vi "Main.vi"(11 "Error in":errorcluster) -> (15 "Error out":errorcluster)   [LabVIEW 2020, in "File explorer 2.0.lvlib"]
doc: "This VI is the expanded implementation of file explorer here this has additional features of adding and getting folder data and copying the selected files form one location to another location"
uses:
  File explorer 2.0.lvlib
  Typedefs/Data Cluster.ctl
  <vilib>/Utility/miscctls.llb/LVPositionTypeDef.ctl
  Typedefs/Queue operations.ctl
panel:
  in  "Stop":bool
  in  "Search":string
  in  "Copy":bool
  in  "Operation":bool
  in  "File input":path
  in  "File system":string(tree)
  out "File details":string
  # "FILE EXPLORER 2.0"
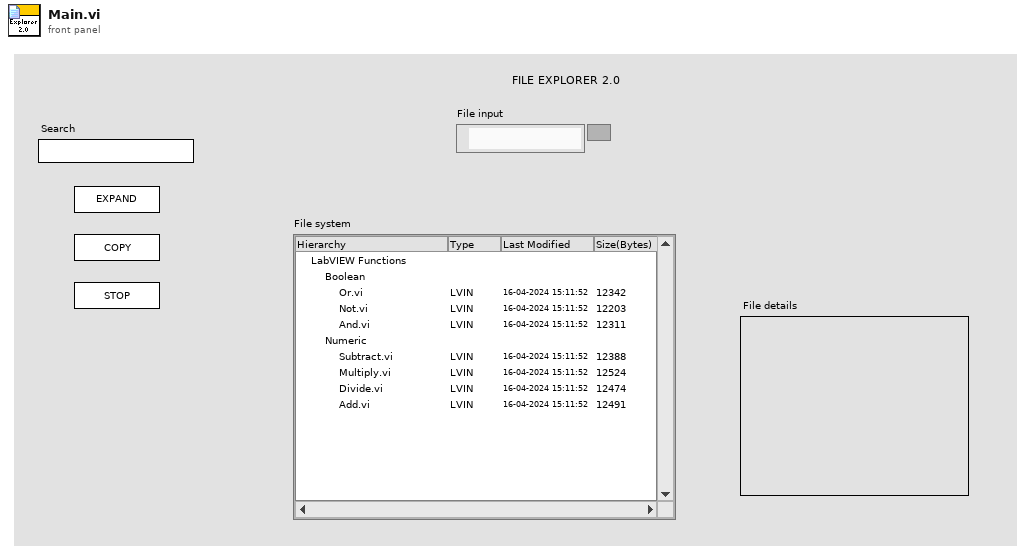
[diagram p1: front panel]
types:
  T1 = typedef "File explorer 2.0.lvlib/Queue operations.ctl" = enum16{"Create", "Enqueue", "Enstack", "Dequeue", "Flush", "Release"}
  T2 = typedef "File explorer 2.0.lvlib/Data Cluster.ctl" = cluster{"Copy":bool, "Operation":bool, "File input":path, "Search":string, "File details":string, "Folder":string[], "Position":T3, "Selected Files":string[], "Reverse":bool}
  T3 = typedef "LVPositionTypeDef.ctl" = cluster{"Left":i32, "Top":i32}
  T4 = typedef "LVPoint32TypeDef.ctl" = cluster{"Horizontal":i32, "Vertical":i32}
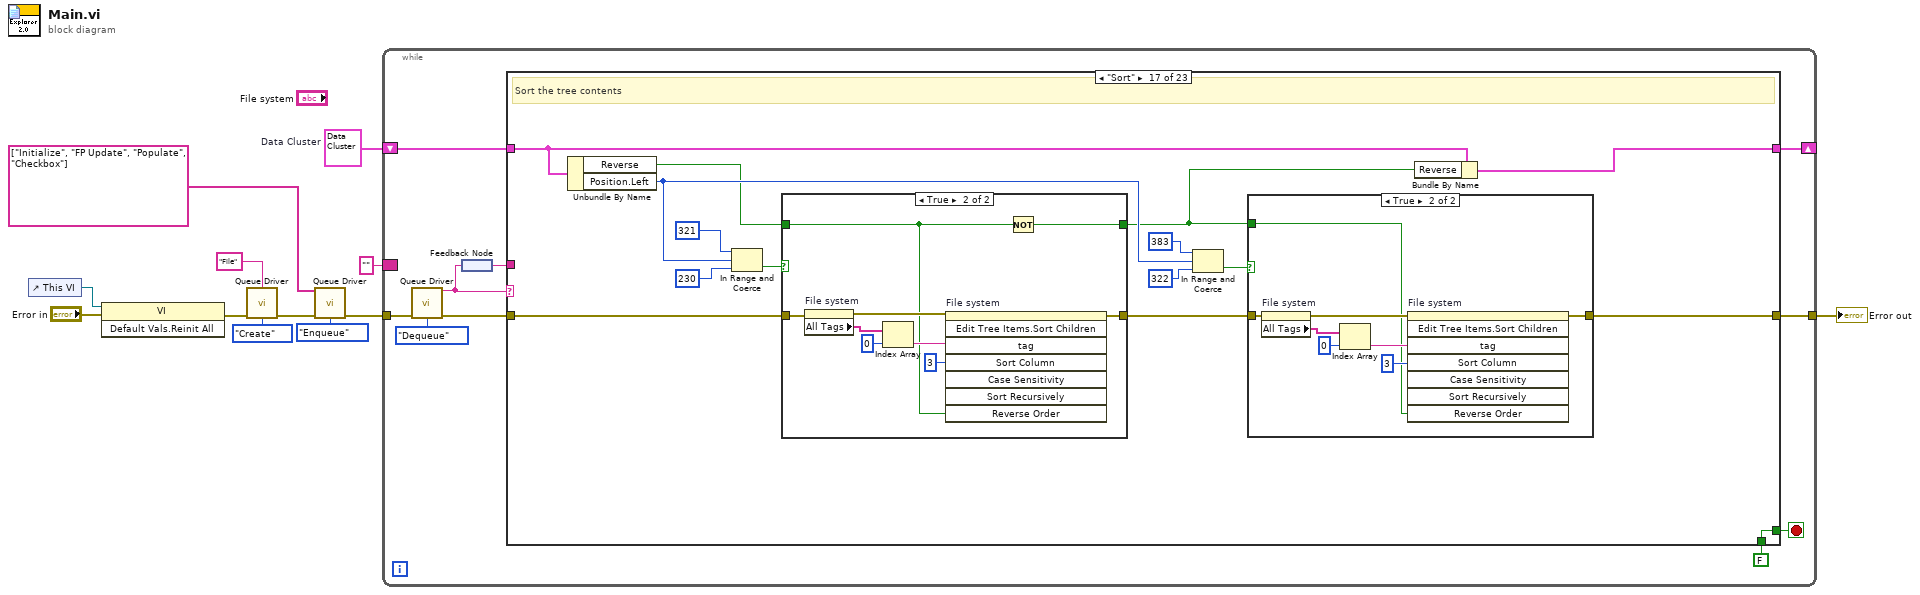
[diagram p0: block diagram]
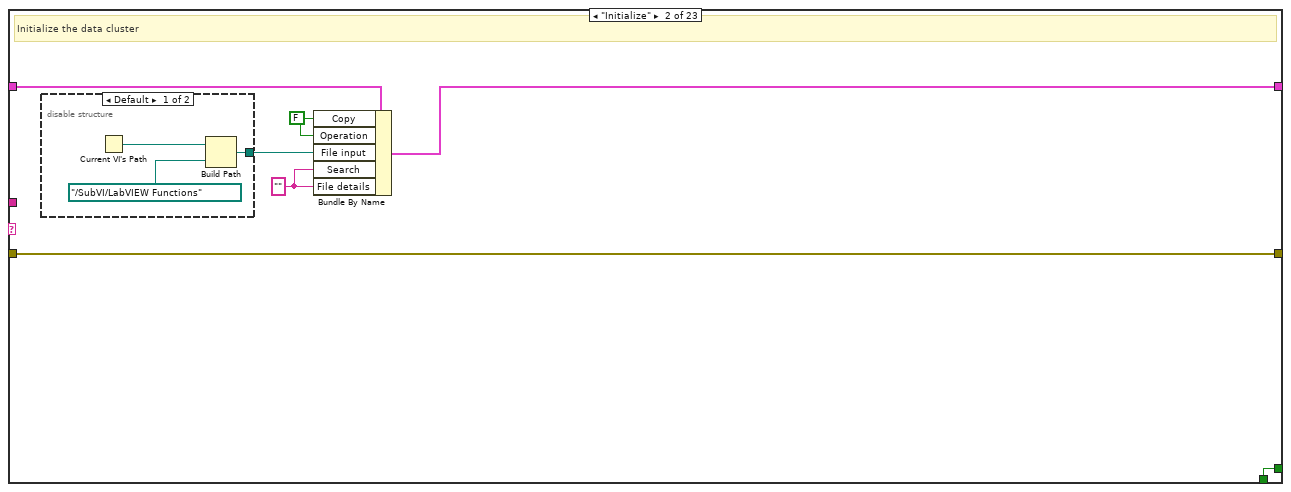
[diagram p3: hidden frame]
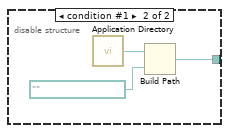
[diagram p4: hidden frame]
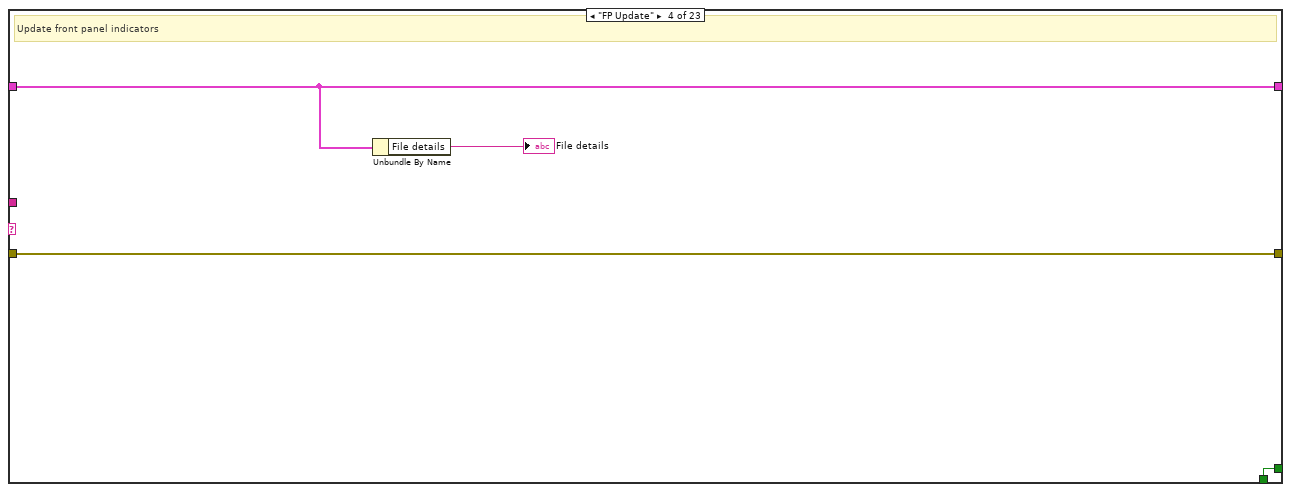
[diagram p6: hidden frame]
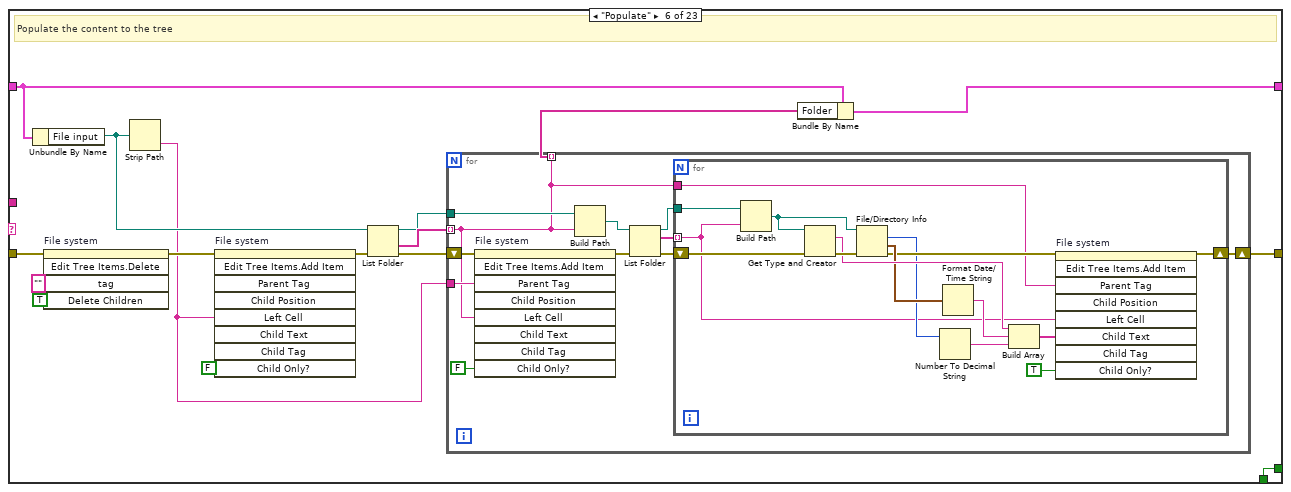
[diagram p8: hidden frame]
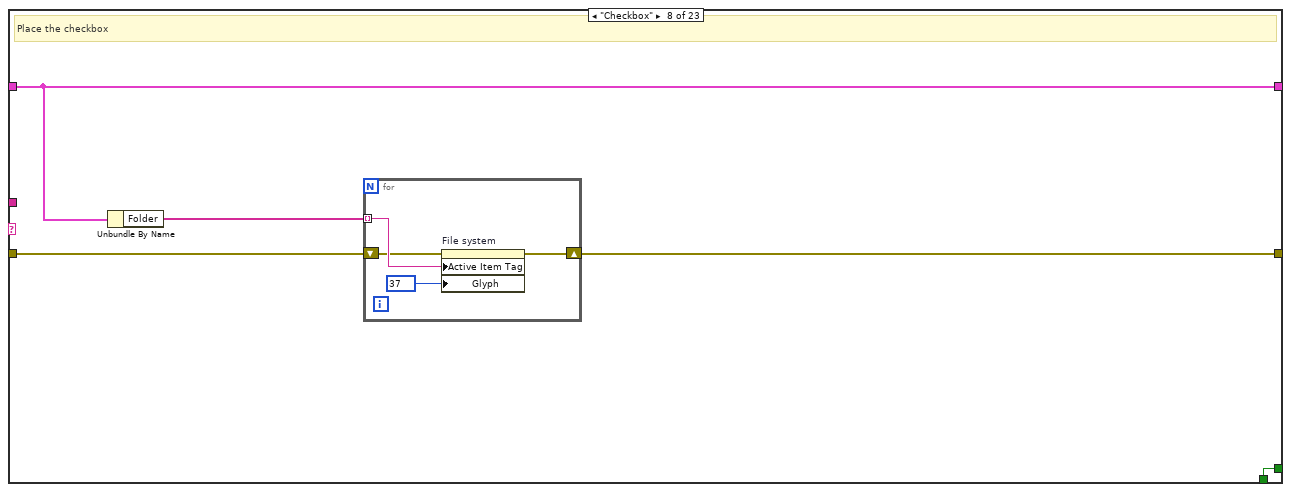
[diagram p10: hidden frame]
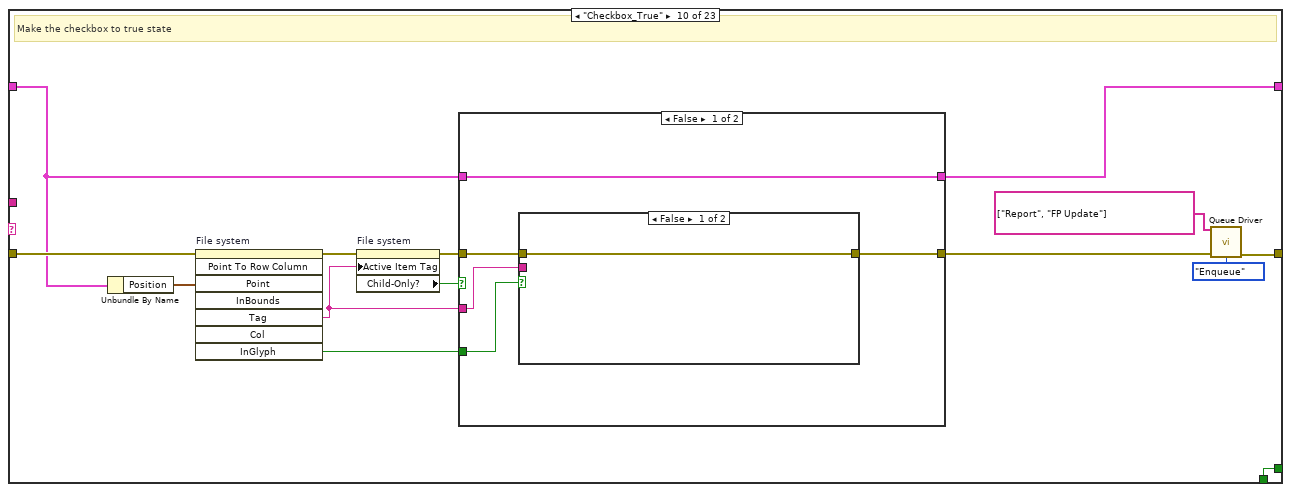
[diagram p12: hidden frame]
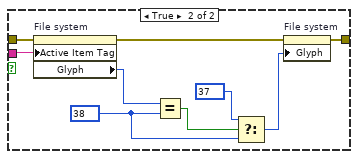
[diagram p13: hidden frame]
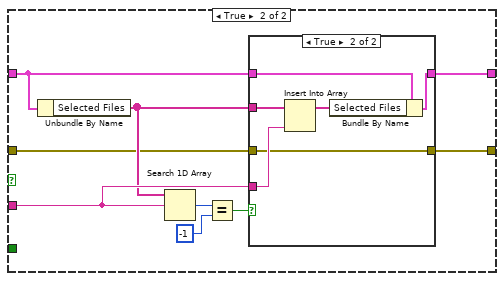
[diagram p14: hidden frame]
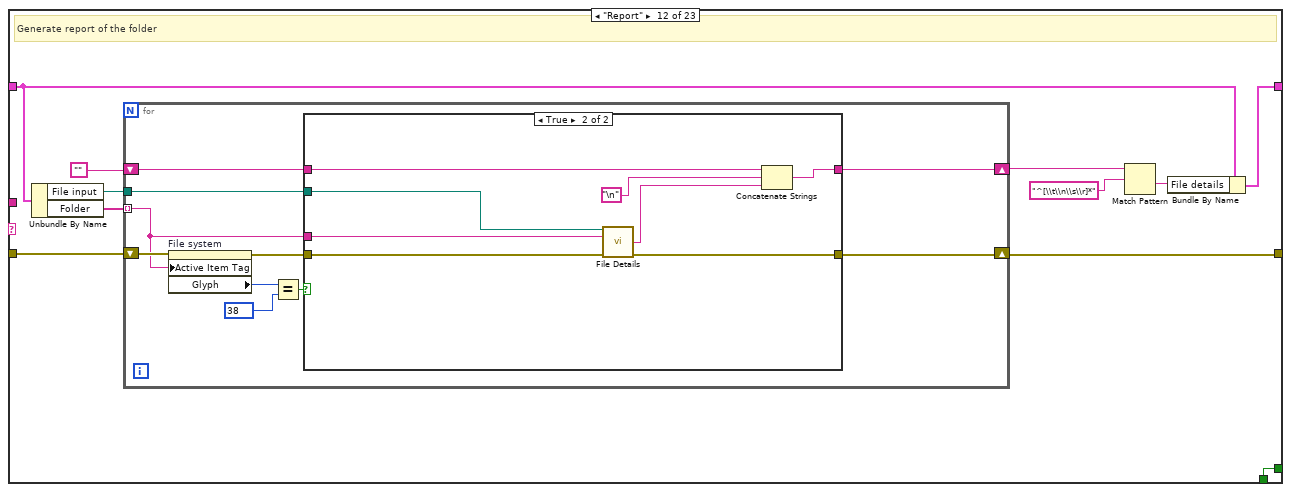
[diagram p17: hidden frame]
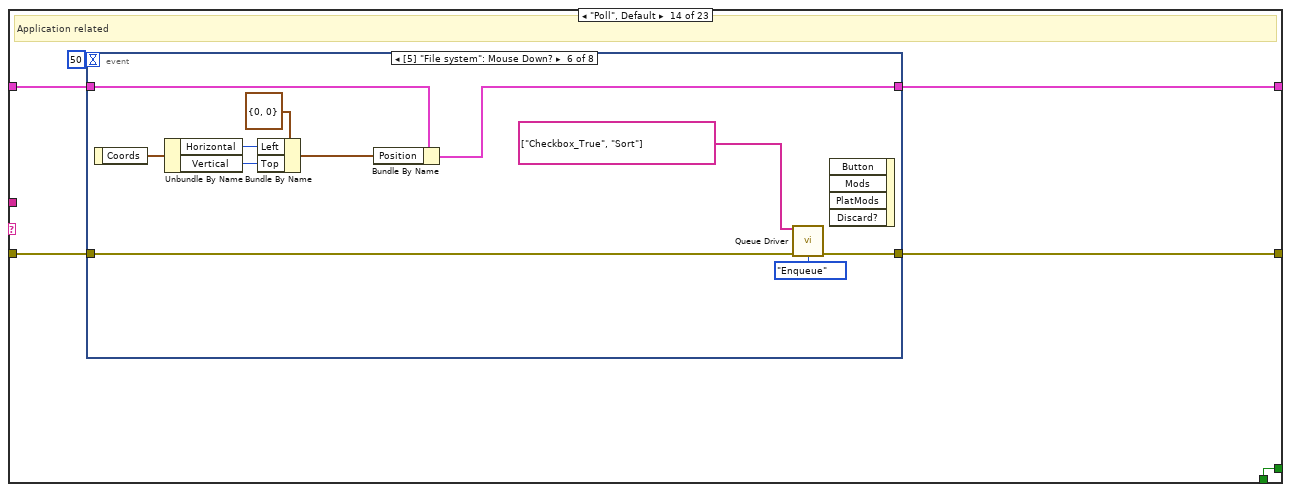
[diagram p20: hidden frame]
diagram:
  w3 = T2 {"Copy"=FALSE, "Operation"=FALSE, "File input"=path "", "Search"="", "File details"="", "Folder"=[], "Position"={"Left"=0, "Top"=0}, "Selected Files"=[], "Reverse"=FALSE}  # Data Cluster
  n1 = control-ref of="This VI"() -> (w12:refnum<vi>)
  n2 = invoke class="VI" method="Default Vals.Reinit All"(reference=w12, error in="Error in") -> (error out=w10:errorcluster)  [unwired: 1 in, 2 out]
  n3 = call "Queue Driver.vi"("Name"="File", "Error in"=w10, "Queue Operations"=Queue_operations."Create") -> ("Error out"=w8:errorcluster)  [unwired: 11 in, 1 out]
  n4 = call "Queue Driver.vi"("Enqueue states"=string[] ["Initialize", "FP Update", "Populate", "Checkbox"], "Error in"=w8, "Queue Operations"=Queue_operations."Enqueue") -> ("Error out"=w6:errorcluster)  [unwired: 11 in, 1 out]
  n5 = while {
    border: "" ("Dequeued state") -> [_]
    tunnel: w6 -> [w20]
    tunnel: [w16] -> w4
    shift-right: [w15] -> _
    shift-left: w3 -> [w14]
    stop <- w22 stop-if-true
    n6 = call "Queue Driver.vi"("Error in"=w20, "Queue Operations"=Queue_operations."Dequeue") -> ("Dequeued state"=w19:string, "Error out"=w17:errorcluster)  [unwired: 12 in]
    n7 = feedback-in #1(w19) -> ()
    n8 = feedback #1() -> (w18:string)
    n9 = case shown="\"Sort\"" w19 {
      tunnel: [w25 w32 w41 w45 w48 w64 w93 w98 w105 w119 w154 w165 w188 w194 w247 w255 w280 w304 w307 w310 w324 w332 TRUE] -> w22
      tunnel: FALSE -> [w25 w32 w41 w45 w48 w64 w93 w98 w105 w119 w154 w165 w188 w194 w247 w255 w280 w304 w307 w310 w324 w332 _]
      tunnel: w18 -> [_ _ _ _ _ _ _ _ _ _ _ _ _ _ _ _ _ _ _ _ w315 _ _]
      tunnel: w17 -> [w24 w31 w40 w44 w47 w63 w92 w96 w104 w118 w153 w164 w187 w191 w246 w254 w276 w303 w306 w309 w311 w331 w337]
      tunnel: [w24 w31 w40 w44 w47 w52 w92 w97 w104 w107 w153 w160 w187 w192 w246 w251 w270 w303 w306 w309 w312 w331 w335] -> w16
      tunnel: [w23 w29 w39 w43 w46 w50 w91 w95 w103 w112 w152 w156 w186 w190 w245 w249 w267 w302 w305 w308 w323 w330 w339] -> w15
      tunnel: w14 -> [w23 w30 w39 w43 w46 w51 w91 w95 w103 w114 w152 w157 w186 w189 w245 w250 w268 w302 w305 w308 w323 w330 w339]
      frame "/***Initialize***/" {
      }
      frame "Initialize" {
        w27 = "" ("File details")
        w28 = FALSE ("Copy")
        # "Initialize the data cluster"
        n10 = disable-structure shown="Default" {
          disable-tunnel: [w33 w37] -> w26
          frame condition #0 (active) {
            n11 = Current VI's Path() -> (path=w35:path)
            n12 = Build Path(base path=w35, name or relative path=path "../SubVI/LabVIEW Functions") -> (appended path=w33:path)
          }
          frame condition #1 {
            n13 = call <vilib>:"Application Directory.vi"() -> ("Application Directory"=w36:path)
            n14 = Build Path(base path=w36, name or relative path=path "") -> (appended path=w37:path)
          }
        }
        n15 = Bundle By Name(cluster=w30, "Copy"=w28, "Operation"=w28, "File input"=w26, "Search"=w27, "File details"=w27) -> (w29:T2)
      }
      frame "/***FP Related***/" {
      }
      frame "FP Update" {
        # "Update front panel indicators"
        n16 = Unbundle By Name(w43) -> ("File details"=→"File details":string)
      }
      frame "/***Populate tree***/" {
      }
      frame "Populate" {
        # "Populate the content to the tree"
        n17 = Unbundle By Name(w51) -> ("File input"=w57:path)
        n18 = invoke on="File system" class="Tree (strict)" method="Edit Tree Items.Delete"(error in=w63, "tag"="" ("Tag"), "Delete Children"=TRUE ("Delete Children?")) -> (error out=w60:errorcluster)  [unwired: 2 in, 4 out]
        n19 = Strip Path(path=w57) -> (name=w54:string)  [unwired: 1 out]
        n20 = invoke on="File system" class="Tree (strict)" method="Edit Tree Items.Add Item"(error in=w60, "Left Cell"=w54, "Child Only?"=FALSE) -> (error out=w58:errorcluster)  [unwired: 6 in, 8 out]
        n21 = List Folder(path=w57, error in=w58) -> (path out=w53:path, folder names=w56:string[], error out=w55:errorcluster)  [unwired: 2 in, 1 out]
        n22 = for {
          tunnel: w56 -> [w65] mode=indexing
          tunnel: w54 -> [w74]
          tunnel: w53 -> [w72]
          shift-right: [w69] -> w52
          shift-left: w55 -> [w75]
          tunnel: [w65] -> w49 mode=indexing
          n23 = invoke on="File system" class="Tree (strict)" method="Edit Tree Items.Add Item"(error in=w75, "Parent Tag"=w74, "Left Cell"=w65, "Child Only?"=FALSE) -> (error out=w70:errorcluster)  [unwired: 5 in, 8 out]
          n24 = Build Path(base path=w72, name or relative path=w65) -> (appended path=w71:path)
          n25 = List Folder(path=w71, error in=w70) -> (path out=w66:path, filenames=w67:string[], error out=w68:errorcluster)  [unwired: 2 in, 1 out]
          n26 = for {
            shift-right: [w90] -> w69
            shift-left: w68 -> [w84]
            tunnel: [w76] -> _ mode=indexing
            tunnel: w67 -> [w76] mode=indexing
            tunnel: w66 -> [w85]
            tunnel: w65 -> [w77]
            n27 = Build Path(base path=w85, name or relative path=w76) -> (appended path=w80:path)
            n28 = Get Type and Creator(4:w84, 7:w80) -> (0:w83:errorcluster, 2:w82:string)  [unwired: 2 out]
            n29 = File/Directory Info(path=w80, error in=w83) -> (size=w78:i64, last mod=w81:timestamp, error out=w79:errorcluster)  [unwired: 4 out]
            n30 = Number To Decimal String(number=w78) -> (decimal integer string=w88:string)  [unwired: 1 in]
            n31 = Format Date/Time String(seconds (now)=w81) -> (date/time string=w86:string)  [unwired: 2 in]
            n32 = Build Array(w82, w86, w88) -> (w87:string[])
            n33 = invoke on="File system" class="Tree (strict)" method="Edit Tree Items.Add Item"(error in=w79, "Parent Tag"=w77, "Left Cell"=w76, "Child Text"=w87, "Child Only?"=TRUE) -> (error out=w90:errorcluster)  [unwired: 4 in, 8 out]
          }
        }
        n34 = Bundle By Name(cluster=w51, "Folder"=w49) -> (w50:T2)
      }
      frame "/***Add Checkbox***/" {
      }
      frame "Checkbox" {
        # "Place the checkbox"
        n35 = Unbundle By Name(w95) -> ("Folder"=w94:string[])
        n36 = for {
          tunnel: w94 -> [w101] mode=indexing
          shift-right: [w102] -> w97
          shift-left: w96 -> [w99]
          n37 = property on="File system" class="Tree (strict)"(error in=w99, "Active Item Tag"=w101, "Glyph"=37) -> (error out=w102:errorcluster)  [unwired: 1 in, 1 out]
        }
      }
      frame "/***Set checkbox to true***/" {
      }
      frame "Checkbox_True" {
        # "Make the checkbox to true state"
        n38 = Unbundle By Name(w114) -> ("Position"=w117:T3)
        n39 = invoke on="File system" class="Tree (strict)" method="Point To Row Column"(error in=w118, "Point"=w117) -> (error out=w116:errorcluster, "Tag"=w113:string, "InGlyph"=w110:bool)  [unwired: 6 in, 5 out]
        n40 = property on="File system" class="Tree (strict)"(error in=w116, "Active Item Tag"=w113) -> (error out=w111:errorcluster, "Child-Only?"=w115:bool)  [unwired: 1 in, 1 out]
        n41 = case shown="False" w115 {
          tunnel: w114 -> [w122 w138]
          tunnel: w113 -> [w123 w140]
          tunnel: [w122 w137] -> w112
          tunnel: w111 -> [w124 w135]
          tunnel: w110 -> [w121 _]
          tunnel: [w120 w136] -> w108
          frame False {
            n42 = case shown="False" w121 {
              tunnel: w124 -> [w125 w134]
              tunnel: w123 -> [_ w133]
              tunnel: [w125 w126] -> w120
              frame False {
              }
              frame True {
                w129 = 38
                n43 = property on="File system" class="Tree (strict)"(error in=w134, "Active Item Tag"=w133) -> (error out=w127:errorcluster, "Glyph"=w131:i32)  [unwired: 1 in, 1 out]
                n44 = Equal?(x=w131, y=w129) -> (x = y?=w130:bool)
                n45 = Select(t=37, s=w130, f=w129) -> (s? t:f=w128:i32)
                n46 = property on="File system" class="Tree (strict)"(error in=w127, "Glyph"=w128) -> (error out=w126:errorcluster)  [unwired: 1 in, 1 out]
              }
            }
          }
          frame True {
            n47 = Unbundle By Name(w138) -> ("Selected Files"=w139:string[])
            n48 = Search 1D Array(1D array=w139, element=w140) -> (index of element=w142:i32)  [unwired: 1 in]
            n49 = Equal?(x=w142, y=-1) -> (x = y?=w141:bool)
            n50 = case shown="True" w141 {
              tunnel: w139 -> [_ w151]
              tunnel: w140 -> [_ w150]
              tunnel: w138 -> [w145 w149]
              tunnel: [w145 w147] -> w137
              tunnel: [w144 w146] -> w136
              tunnel: w135 -> [w144 w146]
              frame False {
              }
              frame True {
                n51 = Insert Into Array(array=w151, new element=w150) -> (w148:string[])  [unwired: 1 in]
                n52 = Bundle By Name(cluster=w149, "Selected Files"=w148) -> (w147:T2)
              }
            }
          }
        }
        n53 = call "Queue Driver.vi"("Enqueue states"=string[] ["Report", "FP Update"], "Error in"=w108, "Queue Operations"=Queue_operations."Enqueue") -> ("Error out"=w107:errorcluster)  [unwired: 11 in, 1 out]
      }
      frame "/***Generate Report***/" {
      }
      frame "Report" {
        # "Generate report of the folder"
        n54 = Unbundle By Name(w157) -> ("File input"=w162:path, "Folder"=w163:string[])
        n55 = for {
          tunnel: w163 -> [w167] mode=indexing
          tunnel: w162 -> [w166]
          shift-right: [w169] -> w158
          shift-left: "" -> [w168]
          shift-right: [w170] -> w160
          shift-left: w164 -> [w175]
          n56 = property on="File system" class="Tree (strict)"(error in=w175, "Active Item Tag"=w167) -> (error out=w171:errorcluster, "Glyph"=w174:i32)  [unwired: 1 in, 1 out]
          n57 = Equal?(x=w174, y=38) -> (x = y?=w172:bool)
          n58 = case shown="True" w172 {
            tunnel: w171 -> [w177 w183]
            tunnel: [w177 w182] -> w170
            tunnel: [w176 w178] -> w169
            tunnel: w168 -> [w176 w185]
            tunnel: w167 -> [_ w181]
            tunnel: w166 -> [_ w180]
            frame False {
            }
            frame True {
              n59 = call "File Details.vi"("Path"=w180, "File/Folder Name"=w181, "Error In"=w183) -> ("Report"=w179:string, "error out"=w182:errorcluster)  [unwired: 11 in]
              n60 = Concatenate Strings(w185, "\n", w179) -> (w178:string)
            }
          }
        }
        n61 = Match Pattern(string=w158, regular expression="^[\\t\\n\\s\\r]*") -> (after substring=w155:string)  [unwired: 1 in, 3 out]
        n62 = Bundle By Name(cluster=w157, "File details"=w155) -> (w156:T2)
      }
      frame "/***Application Related***/" {
      }
      frame "Poll", Default {
        # "Application related"
        n63 = event shown="[5] \"File system\": Mouse Down?" {
          selector: _ -> [_ _ _ _ _ _ _ _]
          dyn-events: _ -> [_ _ _ _ _ _ _ _]
          timeout: 50 -> [_ _ _ _ _ _ _ _]
          tunnel: [w196 w197 w206 w210 w217 w225 w234 w242] -> w192
          tunnel: w191 -> [w196 w198 w207 w211 w218 w226 w235 w243]
          tunnel: [w195 w201 w208 w214 w221 w229 w238 w239] -> w190
          tunnel: w189 -> [w195 w201 w208 w215 w222 w230 w238 w239]
          event Timeout {
            n64 = event-data() -> ()  [unwired: 1 in, 1 out]
          }
          event "Copy": Value Change {
            n65 = event-data() -> ()  [unwired: 1 in, 1 out]
            n66 = call "Queue Driver.vi"("Enqueue states"=string[] ["Copy"], "Error in"=w198, "Queue Operations"=Queue_operations."Enqueue") -> ("Error out"=w197:errorcluster)  [unwired: 11 in, 1 out]
          }
          event "Operation": Value Change {
            n67 = event-data() -> ("NewVal"=w205:bool)  [unwired: 1 in]
            n68 = Select(t=TRUE ("NewVal"), s=w205, f=FALSE ("NewVal")) -> (s? t:f=w202:bool)
            n69 = invoke on="File system" class="Tree (strict)" method="Open/Close.Open/Close All"(error in=w207, "Open"=w202) -> (error out=w206:errorcluster)  [unwired: 2 in, 3 out]
          }
          event "File input": Value Change {
            n70 = event-data() -> ("NewVal"=w213:path)  [unwired: 1 in]
            n71 = call "Queue Driver.vi"("Enqueue states"=string[] ["Populate"], "Error in"=w211, "Queue Operations"=Queue_operations."Enqueue") -> ("Error out"=w210:errorcluster)  [unwired: 11 in, 1 out]
            n72 = Bundle By Name(cluster=w215, "File input"=w213) -> (w214:T2)
          }
          event "Search": Value Change {
            n73 = event-data() -> ("NewVal"=w220:string)  [unwired: 1 in]
            n74 = call "Queue Driver.vi"("Enqueue states"=string[] ["Search"], "Error in"=w218, "Queue Operations"=Queue_operations."Enqueue") -> ("Error out"=w217:errorcluster)  [unwired: 11 in, 1 out]
            n75 = Bundle By Name(cluster=w222, "Search"=w220) -> (w221:T2)
          }
          event "File system": Mouse Down? {
            n76 = event-data() -> ("Coords"=w233:T4)  [unwired: 1 in]
            n77 = Unbundle By Name(w233) -> ("Horizontal"=w223:i32, "Vertical"=w231:i32)
            n78 = Bundle By Name(cluster=T3 {"Left"=0, "Top"=0} ("Point"), "Left"=w223, "Top"=w231) -> (w228:T3)
            n79 = Bundle By Name(cluster=w230, "Position"=w228) -> (w229:T2)
            n80 = call "Queue Driver.vi"("Enqueue states"=string[] ["Checkbox_True", "Sort"], "Error in"=w226, "Queue Operations"=Queue_operations."Enqueue") -> ("Error out"=w225:errorcluster)  [unwired: 11 in, 1 out]
            n81 = event-data() -> ()  [unwired: 5 in, 1 out]
          }
          event "Stop": Value Change {
            n82 = event-data() -> ()  [unwired: 1 in, 1 out]
            n83 = call "Queue Driver.vi"("Enqueue states"=string[] ["Exit"], "Error in"=w235, "Queue Operations"=Queue_operations."Enqueue") -> ("Error out"=w234:errorcluster)  [unwired: 11 in, 1 out]
          }
          event Panel Close? {
            n84 = event-data() -> ()  [unwired: 1 in, 4 out]
            n85 = call "Queue Driver.vi"("Enqueue states"=string[] ["Exit"], "Error in"=w243, "Queue Operations"=Queue_operations."Enqueue") -> ("Error out"=w242:errorcluster)  [unwired: 11 in, 1 out]
            n86 = event-data("Discard?"=TRUE) -> ()  [unwired: 1 in, 1 out]
          }
        }
      }
      frame "/***Copy files***/" {
      }
      frame "Copy" {
        # "Copy files to the specific location"
        n87 = Unbundle By Name(w250) -> ("File input"=w253:path, "Selected Files"=w252:string[])
        n88 = for {
          tunnel: w253 -> [w264]
          tunnel: w252 -> [w262] mode=indexing
          shift-right: [w259] -> w251
          shift-left: w254 -> [w265]
          n89 = invoke on="File system" class="Tree (strict)" method="Navigate Tree.Get Parent"(error in=w265, "tag"=w262) -> (error out=w260:errorcluster, "Navigate Tree:Get Parent"=w263:string)  [unwired: 2 in, 2 out]
          n90 = Build Path(base path=w264, name or relative path=w263) -> (appended path=w261:path)
          n91 = Build Path(base path=w261, name or relative path=w262) -> (appended path=w256:path)
          n92 = Copy(7:"Enter the path" ("prompt (Choose or enter target path for copy)"), 8:w260, 9:TRUE ("overwrite (F)"), 11:w256) -> (0:w259:errorcluster)  [unwired: 1 in, 2 out]
        }
        n93 = Bundle By Name(cluster=w250, "Selected Files"=string[] []) -> (w249:T2)
      }
      frame "Sort" {
        # "Sort the tree contents"
        n94 = Unbundle By Name(w268) -> ("Reverse"=w269:bool, "Position.Left"=w275:i32)
        n95 = In Range and Coerce(upper limit=321, x=w275, lower limit=230) -> (In Range?=w277:bool)  [unwired: 1 out]
        n96 = case shown="True" w277 {
          tunnel: w276 -> [w292 w297]
          tunnel: [w292 w300] -> w271
          tunnel: w269 -> [w291 w293]
          tunnel: [w290 w294] -> w266
          frame False {
            n97 = Not(x=w291) -> (.not. x?=w290:bool)
          }
          frame True {
            n98 = property on="File system" class="Tree (strict)"(error in=w297) -> (error out=w296:errorcluster, "All Tags"=w299:string[])  [unwired: 1 in, 1 out]
            n99 = Index Array(array=w299, index=0) -> (element=w295:string)
            n100 = invoke on="File system" class="Tree (strict)" method="Edit Tree Items.Sort Children"(error in=w296, "tag"=w295, "Sort Column"=3, "Reverse Order"=w293) -> (error out=w300:errorcluster)  [unwired: 4 in, 7 out]
            n101 = Not(x=w293) -> (.not. x?=w294:bool)
          }
        }
        n102 = In Range and Coerce(upper limit=383, x=w275, lower limit=322) -> (In Range?=w272:bool)  [unwired: 1 out]
        n103 = case shown="True" w272 {
          tunnel: w271 -> [w281 w287]
          tunnel: [w281 w288] -> w270
          tunnel: w266 -> [_ w282]
          frame False {
          }
          frame True {
            n104 = property on="File system" class="Tree (strict)"(error in=w287) -> (error out=w286:errorcluster, "All Tags"=w285:string[])  [unwired: 1 in, 1 out]
            n105 = Index Array(array=w285, index=0) -> (element=w283:string)
            n106 = invoke on="File system" class="Tree (strict)" method="Edit Tree Items.Sort Children"(error in=w286, "tag"=w283, "Sort Column"=3, "Reverse Order"=w282) -> (error out=w288:errorcluster)  [unwired: 4 in, 7 out]
          }
        }
        n107 = Bundle By Name(cluster=w268, "Reverse"=w266) -> (w267:T2)
      }
      frame "/***Search***/" {
      }
      frame "Search" {
        # "Highlight the item selected"
      }
      frame "/***Handle Error***/" {
      }
      frame "Error" {
        # "Handle the errors"
        n108 = Unbundle By Name(w311) -> ("code"=w320:i32, "source"=w319:string)
        n109 = call <vilib>:"Clear Errors.vi"("error in (no error)"=w311, "specific error code to clear (0: all)"=w320) -> ("error out"=w322:errorcluster)  [unwired: 4 in, 1 out]
        n110 = Format Into String(format string="Error occurred in state \"%s\"!!\nError Code: %d\nError Source: %s\n\nDo you wish to continue?", error in=w322, w315, w320, w319) -> (resulting string=w318:string, error out=w313:errorcluster)  [unwired: 1 in]
        n111 = Two Button Dialog(message=w318, 1:"Exit" ("F button name (\"Cancel\")"), 2:"Continue" ("T button name (\"OK\")")) -> (T button?=w314:bool)
        n112 = case shown="False" w314 {
          tunnel: w313 -> [w325 w328]
          tunnel: [w325 w326] -> w312
          frame False {
            # "Continue"
          }
          frame True {
            # "Exit"
            n113 = call "Queue Driver.vi"("Enqueue states"=string[] ["Exit"], "Error in"=w328, "Queue Operations"=Queue_operations."Enqueue") -> ("Error out"=w326:errorcluster)  [unwired: 11 in, 1 out]
          }
        }
      }
      frame "/***Exit***/" {
      }
      frame "Exit" {
        # "Flush and Release the queue"
        # "Terminate execution of the system"
        n114 = call "Queue Driver.vi"("Error in"=w337, "Queue Operations"=Queue_operations."Flush") -> ("Error out"=w336:errorcluster)  [unwired: 12 in, 1 out]
        n115 = call "Queue Driver.vi"("Error in"=w336, "Queue Operations"=Queue_operations."Release") -> ("Error out"=w335:errorcluster)  [unwired: 12 in, 1 out]
      }
    }
  }
  "Error out" <- w4
